vi "Record Filesize.vi"(6 "No file limit":bool, 8 "error in (no error)":errorcluster, 9 "BaseSize":u16(ring) items=["KiloSamples", "MegaSamples", "GigaSamples"], 10 "Filesize":i32, 11 "VISA resource name":refnum<visa-resource-name>) -> (0 "error out":errorcluster, 3 "VISA resource name out":refnum<visa-resource-name>)   [LabVIEW 2017, in "Sefram DAS220.lvlib"]
doc: "Set record filesize."
uses:
  <instrlib>/Sefram DAS220/Sefram DAS220.lvlib
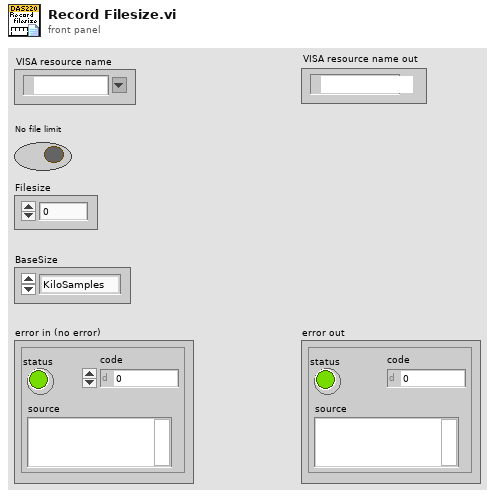
[diagram p1: front panel]
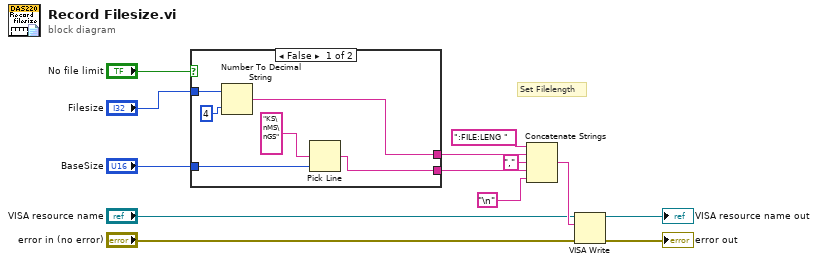
[diagram p0: block diagram]
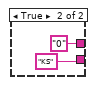
[diagram p2: hidden frame]
diagram:
  # "Set Filelength"
  n1 = case shown="False" "No file limit" {
    tunnel: "Filesize" -> [w19 _]
    tunnel: [w16 "0"] -> w4
    tunnel: [w15 "KS" ("output string")] -> w3
    tunnel: "BaseSize" -> [w14 _]
    frame False {
      n2 = Number To Decimal String(number=w19, width (-)=i16 4) -> (decimal integer string=w16:string)
      n3 = Pick Line(multi-line string="KS\nMS\nGS", line index=w14) -> (output string=w15:string)  [unwired: 1 in]
    }
    frame True {
    }
  }
  n4 = Concatenate Strings(":FILE:LENG " ("string"), w4, "," ("string"), w3, "\n") -> (w13:string)
  n5 = VISA Write(VISA resource name="VISA resource name", write buffer=w13, error in (no error)="error in (no error)") -> (VISA resource name out=→"VISA resource name out":refnum<visa-resource-name>, error out=→"error out":errorcluster)  [unwired: 1 out]
